vi "主板信息可变参数配置.vi"(11 "从板个数":dbl) -> (0 "主板温度起始值":string[](array[string]), 1 "主板温度个数":string[](array[string]), 2 "主板电压起始值":string[](array[string]), 3 "电池节数":string[](array[string]))   [LabVIEW 2013]
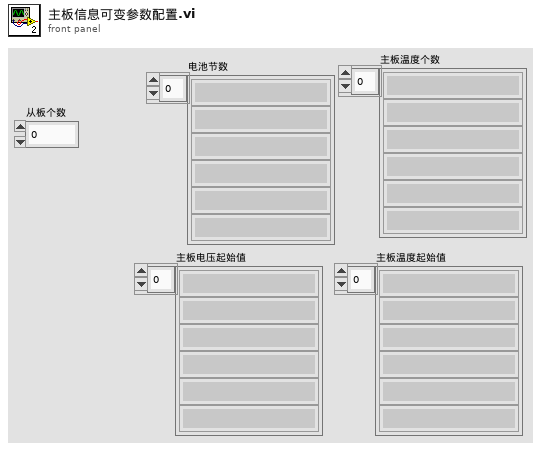
[diagram p1: front panel]
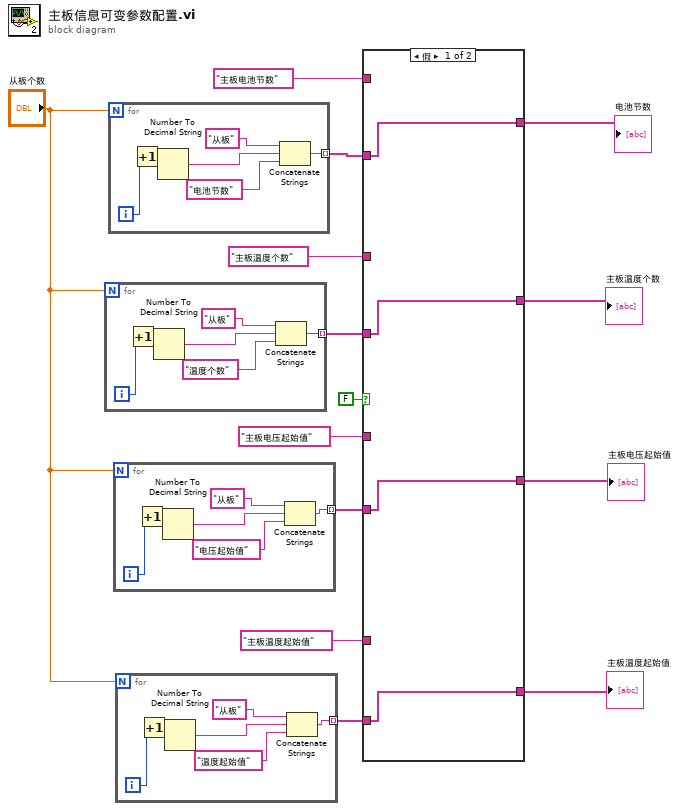
[diagram p0: block diagram]
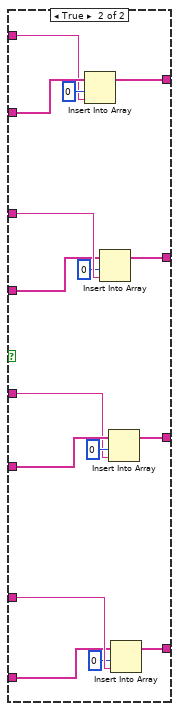
[diagram p2: hidden frame]
diagram:
  n1 = for {
    N: "从板个数" -> [_]
    tunnel: [w15] -> w10 mode=indexing
    i -> [w20]
    n2 = Increment(x=w20) -> (x+1=w19:i32)
    n3 = Number To Decimal String(number=w19) -> (decimal integer string=w17:string)  [unwired: 1 in]
    n4 = Concatenate Strings("从板", w17, "温度个数") -> (w15:string)
  }
  n5 = for {
    N: "从板个数" -> [_]
    tunnel: [w21] -> w13 mode=indexing
    i -> [w26]
    n6 = Increment(x=w26) -> (x+1=w25:i32)
    n7 = Number To Decimal String(number=w25) -> (decimal integer string=w23:string)  [unwired: 1 in]
    n8 = Concatenate Strings("从板", w23, "电池节数") -> (w21:string)
  }
  n9 = for {
    N: "从板个数" -> [_]
    tunnel: [w27] -> w7 mode=indexing
    i -> [w32]
    n10 = Increment(x=w32) -> (x+1=w31:i32)
    n11 = Number To Decimal String(number=w31) -> (decimal integer string=w29:string)  [unwired: 1 in]
    n12 = Concatenate Strings("从板", w29, "电压起始值") -> (w27:string)
  }
  n13 = for {
    N: "从板个数" -> [_]
    tunnel: [w33] -> w4 mode=indexing
    i -> [w38]
    n14 = Increment(x=w38) -> (x+1=w37:i32)
    n15 = Number To Decimal String(number=w37) -> (decimal integer string=w35:string)  [unwired: 1 in]
    n16 = Concatenate Strings("从板", w35, "温度起始值") -> (w33:string)
  }
  n17 = case shown="假" FALSE {
    tunnel: [w42 w58] -> w14
    tunnel: w13 -> [w42 w56]
    tunnel: "主板电池节数" -> [_ w55]
    tunnel: "主板温度个数" -> [_ w54]
    tunnel: w10 -> [w41 w53]
    tunnel: [w41 w51] -> w9
    tunnel: [w40 w50] -> w8
    tunnel: w7 -> [w40 w48]
    tunnel: "主板电压起始值" -> [_ w47]
    tunnel: "主板温度起始值" -> [_ w46]
    tunnel: w4 -> [w39 w45]
    tunnel: [w39 w43] -> w3
    frame False {
    }
    frame True {
      n18 = Insert Into Array(array=w56, index=0 ("索引"), new element=w55) -> (w58:string[])
      n19 = Insert Into Array(array=w53, index=0 ("索引"), new element=w54) -> (w51:string[])
      n20 = Insert Into Array(array=w48, index=0 ("索引"), new element=w47) -> (w50:string[])
      n21 = Insert Into Array(array=w45, index=0 ("索引"), new element=w46) -> (w43:string[])
    }
  }
  "电池节数" <- w14
  "主板温度个数" <- w9
  "主板电压起始值" <- w8
  "主板温度起始值" <- w3
